vi "VCS Get Analog Input Voltage.vi"(8 "error in (no error)":errorcluster, 10 "number":u16=1, 11 "axis in":cluster{"keyHandle":u32, "nodeId":u16}={"keyHandle"=0, "nodeId"=1}) -> (0 "error out":errorcluster, 2 "voltageValue":i32, 3 "axis out":cluster{"keyHandle":u32, "nodeId":u16}={"keyHandle"=0, "nodeId"=1})   [LabVIEW 2019, in "maxonEPOS.lvlib"]
doc: "<B>VCS Get Analog Input</B> returns the analog value from selected input."
uses:
  Examples/maxonEPOS.lvlib
  Resources/EposCmd64.dll
  Resources/EposCmd.dll
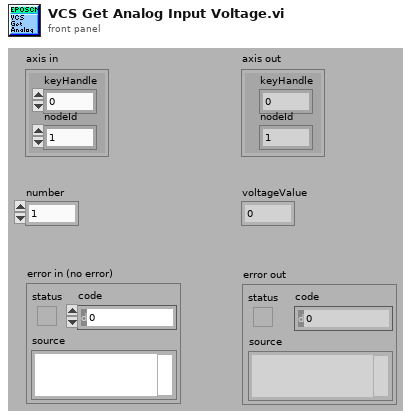
[diagram p1: front panel]
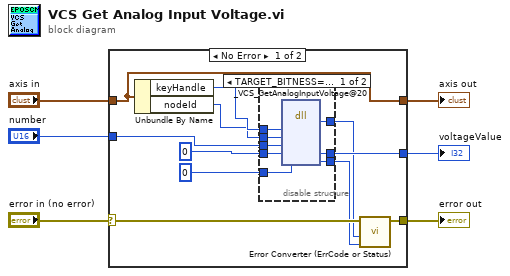
[diagram p0: block diagram]
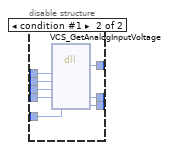
[diagram p2: hidden frame]
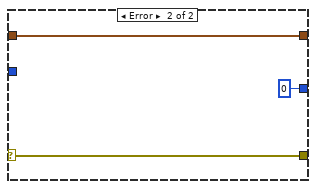
[diagram p3: hidden frame]
diagram:
  n1 = case shown="No Error" "error in (no error)" {
    selector: "error in (no error)" -> [w15 w36]
    tunnel: [w14 w36] -> w5
    tunnel: "number" -> [w17 _]
    tunnel: [w16 u16 0 ("pAnalog")] -> w3
    tunnel: "axis in" -> [w8 w35]
    tunnel: [w8 w35] -> w1
    frame No Error {
      n2 = Unbundle By Name(w8) -> ("keyHandle"=w12:u32, "nodeId"=w11:u16)
      n3 = disable-structure shown="TARGET_BITNESS==32, Standard" {
        disable-tunnel: w17 -> [w25 w33]
        disable-tunnel: [w24 w32] -> w16
        disable-tunnel: [w23 w31] -> w13
        disable-tunnel: w12 -> [w22 w30]
        disable-tunnel: w11 -> [w21 w29]
        disable-tunnel: u16 0 ("pAnalog") -> [w20 w28]
        disable-tunnel: u32 0 ("pErrorCode") -> [w19 w27]
        disable-tunnel: [w18 w26] -> w7
        frame condition #0 (active) {
          n4 = dll-call lib="C:/workspace/project/scancon/sw/SSI_Tool/InstrumentsInterfaces/Motordriver/maxon EPOS/Resources/EposCmd.*" fn="_VCS_GetAnalogInputVoltage@20" ("EposCmd.dll:_VCS_GetAnalogInput@20")("KeyHandle"=w22, "NodeId"=w21, "Number"=w25, "pVoltageValue"=w20, "pErrorCode"=w19) -> ("Rückgabetyp"=w18:i32, "pVoltageValue"=w24:i32, "pErrorCode"=w23:u32)  [unwired: 6 in, 2 out]
        }
        frame condition #1 {
          n5 = dll-call lib="C:/Sources/LabView/maxon EPOS/Resources/EposCmd64.*" fn="VCS_GetAnalogInputVoltage" ("EposCmd.dll:_VCS_GetAnalogInput@20")("KeyHandle"=w30, "NodeId"=w29, "Number"=w33, "pVoltageValue"=w28, "pErrorCode"=w27) -> ("Rückgabetyp"=w26:i32, "pVoltageValue"=w32:i32, "pErrorCode"=w31:u32)  [unwired: 6 in, 2 out]
        }
      }
      n6 = call "Error Converter (ErrCode or Status).vi"("error code"=w13, "return type"=w7, "error in (no error)"=w15) -> ("error out"=w14:errorcluster)  [unwired: 7 in]
    }
    frame Error {
    }
  }
  "voltageValue" <- w3
  "error out" <- w5
  "axis out" <- w1
